vi "Read Exe Version.vi"(10 "beta?":bool, 11 "Application name":path=path "INC.exe") -> (0 "Build Date":string, 1 "Application Path out":path, 2 "Title String":string, 3 "FileVersion":string)   [LabVIEW 2024]
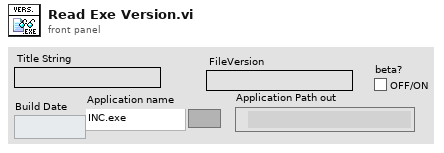
[diagram p1: front panel]
types:
  T1 = enum32{"invalid app kind", "Development System", "Run Time System", "Student Edition", "Embedded LabVIEW", "Evaluation", "Custom"}
  T2 = typedef "FileVersionInformation.ctl" = cluster{"FileVersion":string, "ProductName":string, "InternalName":string, "CompanyName":string, "LegalCopyright":string, "FileDescription":string}
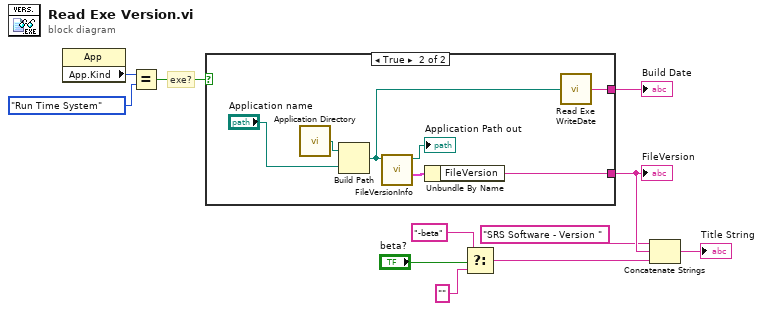
[diagram p0: block diagram]
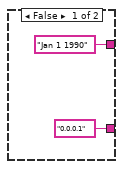
[diagram p2: hidden frame]
diagram:
  # "exe?"
  n1 = property class="App"() -> ("App.Kind"=w8:T1)  [unwired: 2 in, 2 out]
  n2 = Equal?(x=w8, y=T1."Run Time System" ("Application:Kind")) -> (x = y?=w10:bool)
  n3 = case shown="True" w10 {
    tunnel: ["0.0.0.1" ("FileVersion") w19] -> w11
    tunnel: ["Jan 1 1990" ("Last Write Time") w15] -> w5
    frame False {
    }
    frame True {
      n4 = call <vilib>:"Application Directory.vi"() -> ("Application Directory"=w18:path)
      n5 = Build Path(base path=w18, name or relative path="Application name") -> (appended path=w16:path)
      n6 = call <vilib>:"FileVersionInfo.vi"("Application Path in"=w16) -> ("FileVersionInfo Out"=w20:T2, "Application Path out"=→"Application Path out":path)  [unwired: 7 in, 2 out]
      n7 = Unbundle By Name(w20) -> ("FileVersion"=w19:string)
      n8 = call "Read Exe WriteDate.vi"("File Path in"=w16) -> ("Last Write Time"=w15:string)
    }
  }
  "FileVersion" <- w11
  "Build Date" <- w5
  n9 = Select(t="-beta" ("Version"), s="beta?", f="") -> (s? t:f=w4:string)
  n10 = Concatenate Strings("SRS Software - Version " ("Version"), w11, w4) -> (→"Title String":string)
